vi "S4GUI.vi"(7 "Tab ObsEng":enum32{"Obs", "CCD modes", "Eng"}(tab)) -> ()   [LabVIEW 2018] (continued)
                n2555 = call "Write section_name.vi"("error in (no error)"=w5423, "section_name"="CCD_ACS3", "Channel in"=w5424) -> ("error out"=w5422:errorcluster, "Channel out"=w5427:refnum<class "Channel.lvclass">)  [unwired: 7 in]
                n2556 = call-dynamic "save config.vi"("error in (no error)"=w5422, "file config"="lastsaved.cfg", "Channel in"=w5427) -> ("error out"=w5390:errorcluster, "Channel out"=w5392:refnum<class "Channel.lvclass">)  [unwired: 7 in]
                n2557 = local read "Filter3"() -> (w5408:u8)
                n2558 = call-dynamic "Write Filter.vi"("error in (no error)"=w5390, "Filter"=w5408, "Channel in"=w5392) -> ("error out"=w5401:errorcluster, "Channel out"=w5400:refnum<class "Channel.lvclass">)  [unwired: 7 in]
                n2559 = call-dynamic "Read Interface.vi"("error in (no error)"=w5401, "Channel in"=w5400) -> ("error out"=w5403:errorcluster, "Interface.lvclass"=w5398:refnum<class "Interface.lvclass">, "Channel out"=w5399:refnum<class "Channel.lvclass">)  [unwired: 7 in]
                n2560 = call-dynamic "Write Suffix.vi"("error in (no error)"=w5403, "Suffix"=w5384, "Interface in"=w5398) -> ("error out"=w5407:errorcluster, "Interface out"=w5397:refnum<class "Interface.lvclass">)  [unwired: 7 in]
                n2561 = call-dynamic "Write ObsType.vi"("error in (no error)"=w5407, "ObsType"=w5383, "Interface in"=w5397) -> ("error out"=w5406:errorcluster, "Interface out"=w5396:refnum<class "Interface.lvclass">)  [unwired: 7 in]
                n2562 = call-dynamic "Write Object.vi"("error in (no error)"=w5406, "Object"=w5386, "Interface in"=w5396) -> ("error out"=w5405:errorcluster, "Interface out"=w5395:refnum<class "Interface.lvclass">)  [unwired: 7 in]
                n2563 = call-dynamic "Write Comments.vi"("error in (no error)"=w5405, "Comments"=w5387, "Interface in"=w5395) -> ("error out"=w5404:errorcluster, "Interface out"=w5394:refnum<class "Interface.lvclass">)  [unwired: 7 in]
                n2564 = call-dynamic "Write Observer.vi"("error in (no error)"=w5404, "Observer"=w5388, "Interface in"=w5394) -> ("error out"=w5402:errorcluster, "Interface out"=w5393:refnum<class "Interface.lvclass">)  [unwired: 7 in]
                n2565 = call-dynamic "Write Interface.vi"("error in (no error)"=w5402, "Interface.lvclass"=w5393, "Channel in"=w5399) -> ("error out"=w5389:errorcluster, "Channel out"=w5391:refnum<class "Channel.lvclass">)  [unwired: 7 in]
                n2566 = call-dynamic "Read State Machine.vi"("error in (no error)"=w5389, "Device in"=w5391) -> ("error out"=w5355:errorcluster, "State Machine.lvclass"=w5357:refnum<class "State Machine.lvclass">, "Device out"=w5428:refnum<class "Channel.lvclass">)  [unwired: 7 in]
                n2567 = call-dynamic "Read ref StatesQueue.vi"("error in (no error)"=w5355, "State Machine in"=w5357) -> ("error out"=w5362:errorcluster, "ref StatesQueue"=w5361:refnum<queue>, "State Machine out"=w5358:refnum<class "State Machine.lvclass">)  [unwired: 7 in]
                n2568 = Flush Queue(queue=w5361, error in (no error)=w5362) -> (queue out=w5363:refnum<queue>, error out=w5367:errorcluster)  [unwired: 1 out]
                n2569 = Enqueue Element(queue=w5363, element=u32 300 ("State"), error in (no error)=w5367) -> (queue out=w5364:refnum<queue>, error out=w5368:errorcluster)  [unwired: 1 in, 1 out]
                n2570 = Enqueue Element(queue=w5364, element=u32 60 ("State"), error in (no error)=w5368) -> (queue out=w5365:refnum<queue>, error out=w5366:errorcluster)  [unwired: 1 in, 1 out]
                n2571 = call-dynamic "Write ref StatesQueue.vi"("error in (no error)"=w5366, "ref StatesQueue"=w5365, "State Machine in"=w5358) -> ("error out"=w5354:errorcluster, "State Machine out"=w5356:refnum<class "State Machine.lvclass">)  [unwired: 7 in]
                n2572 = call-dynamic "Write State.vi"("error in (no error)"=w5354, "State"=0, "State Machine in"=w5356) -> ("error out"=w5420:errorcluster, "State Machine out"=w5429:refnum<class "State Machine.lvclass">)  [unwired: 7 in]
                n2573 = call-dynamic "Write State Machine.vi"("error in (no error)"=w5420, "State Machine.lvclass"=w5429, "Device in"=w5428) -> ("error out"=w5431:errorcluster, "Device out"=w5430:refnum<class "Channel.lvclass">)  [unwired: 7 in]
                n2574 = call-dynamic "Write Channel.vi"("error in (no error)"=w5431, "Channel.lvclass"=w5430, "Acquisition in"=w5413) -> ("error out"=w5409:errorcluster, "Acquisition out"=w5410:refnum<class "Acquisition.lvclass">)  [unwired: 7 in]
              }
            }
            n2575 = case shown="True" w5243 {
              tunnel: w5245 -> [w5267 w5326]
              tunnel: w5244 -> [w5266 w5325]
              tunnel: [w5267 w5324] -> w5259
              tunnel: [w5266 w5323] -> w5258
              tunnel: w5236 -> [_ w5302]
              tunnel: w5235 -> [_ w5301]
              tunnel: w5234 -> [_ w5300]
              tunnel: w5233 -> [_ w5298]
              tunnel: w5232 -> [_ w5297]
              frame False {
              }
              frame True {
                # "nome do arquivo .cfg"
                # "seção no arquivo .cfg"
                n2576 = call-dynamic "Read Channel.vi"("error in (no error)"=w5325, "Acquisition in"=w5326) -> ("error out"=w5343:errorcluster, "Channel.lvclass"=w5344:refnum<class "Channel.lvclass">, "Acquisition out"=w5345:refnum<class "Acquisition.lvclass">)  [unwired: 7 in]
                n2577 = call-dynamic "Read Interface.vi"("error in (no error)"=w5343, "Channel in"=w5344) -> ("error out"=w5295:errorcluster, "Interface.lvclass"=w5294:refnum<class "Interface.lvclass">, "Channel out"=w5291:refnum<class "Channel.lvclass">)  [unwired: 7 in]
                n2578 = call-dynamic "Write restoreExpTime.vi"("error in (no error)"=w5295, "restoreExpTime"=TRUE, "Interface in"=w5294) -> ("error out"=w5288:errorcluster, "Interface out"=w5293:refnum<class "Interface.lvclass">)  [unwired: 7 in]
                n2579 = call-dynamic "Read target cluster.vi"("error in (no error)"=w5288, "Channel in"=w5291) -> ("error out"=w5287:errorcluster, "target cluster"=w5289:T30, "Channel out"=w5290:refnum<class "Channel.lvclass">)  [unwired: 7 in]
                n2580 = stacked-sequence {
                  tunnel: w5289 -> [_ w5351]
                  tunnel: [_ w5350] -> w5285
                  tunnel: w5289 -> [w5347 _]
                  tunnel: [w5346 _] -> w5299
                  frame #0 {
                    n2581 = Unbundle By Name(w5347) -> ("FRAME_TRANSFER"=w5346:bool)
                  }
                  frame #1 {
                    # "closed"
                    n2582 = Bundle By Name(cluster=w5351, "SHUTTER_MODE"=u8 2, "FRAME_TRANSFER"=FALSE) -> (w5350:T30)
                  }
                }
                n2583 = call-dynamic "Write PREV_FT.vi"("error in (no error)"=w5287, "PREV_FT"=w5299, "Interface in"=w5293) -> ("error out"=w5286:errorcluster, "Interface out"=w5292:refnum<class "Interface.lvclass">)  [unwired: 7 in]
                n2584 = call-dynamic "Write target cluster.vi"("error in (no error)"=w5286, "target cluster"=w5285, "Channel in"=w5290) -> ("error out"=w5284:errorcluster, "Channel out"=w5283:refnum<class "Channel.lvclass">)  [unwired: 7 in]
                n2585 = Flatten To String(anything=w5285, error in (no error)=w5284) -> (data string=w5342:string, error out=w5341:errorcluster)  [unwired: 2 in, 1 out]
                n2586 = call "Write flatted cluster.vi"("error in (no error)"=w5341, "flatted cluster"=w5342, "Interface in"=w5292) -> ("error out"=w5339:errorcluster, "Interface out"=w5340:refnum<class "Interface.lvclass">)  [unwired: 7 in]
                n2587 = call-dynamic "Write Interface.vi"("error in (no error)"=w5339, "Interface.lvclass"=w5340, "Channel in"=w5283) -> ("error out"=w5335:errorcluster, "Channel out"=w5334:refnum<class "Channel.lvclass">)  [unwired: 7 in]
                n2588 = call "Write section_name.vi"("error in (no error)"=w5335, "section_name"="CCD_ACS4", "Channel in"=w5334) -> ("error out"=w5336:errorcluster, "Channel out"=w5331:refnum<class "Channel.lvclass">)  [unwired: 7 in]
                n2589 = call-dynamic "save config.vi"("error in (no error)"=w5336, "file config"="lastsaved.cfg", "Channel in"=w5331) -> ("error out"=w5305:errorcluster, "Channel out"=w5306:refnum<class "Channel.lvclass">)  [unwired: 7 in]
                n2590 = local read "Filter4"() -> (w5322:u8)
                n2591 = call-dynamic "Write Filter.vi"("error in (no error)"=w5305, "Filter"=w5322, "Channel in"=w5306) -> ("error out"=w5315:errorcluster, "Channel out"=w5314:refnum<class "Channel.lvclass">)  [unwired: 7 in]
                n2592 = call-dynamic "Read Interface.vi"("error in (no error)"=w5315, "Channel in"=w5314) -> ("error out"=w5317:errorcluster, "Interface.lvclass"=w5312:refnum<class "Interface.lvclass">, "Channel out"=w5313:refnum<class "Channel.lvclass">)  [unwired: 7 in]
                n2593 = call-dynamic "Write Suffix.vi"("error in (no error)"=w5317, "Suffix"=w5298, "Interface in"=w5312) -> ("error out"=w5321:errorcluster, "Interface out"=w5311:refnum<class "Interface.lvclass">)  [unwired: 7 in]
                n2594 = call-dynamic "Write ObsType.vi"("error in (no error)"=w5321, "ObsType"=w5297, "Interface in"=w5311) -> ("error out"=w5320:errorcluster, "Interface out"=w5310:refnum<class "Interface.lvclass">)  [unwired: 7 in]
                n2595 = call-dynamic "Write Object.vi"("error in (no error)"=w5320, "Object"=w5300, "Interface in"=w5310) -> ("error out"=w5319:errorcluster, "Interface out"=w5309:refnum<class "Interface.lvclass">)  [unwired: 7 in]
                n2596 = call-dynamic "Write Comments.vi"("error in (no error)"=w5319, "Comments"=w5301, "Interface in"=w5309) -> ("error out"=w5318:errorcluster, "Interface out"=w5308:refnum<class "Interface.lvclass">)  [unwired: 7 in]
                n2597 = call-dynamic "Write Observer.vi"("error in (no error)"=w5318, "Observer"=w5302, "Interface in"=w5308) -> ("error out"=w5316:errorcluster, "Interface out"=w5307:refnum<class "Interface.lvclass">)  [unwired: 7 in]
                n2598 = call-dynamic "Write Interface.vi"("error in (no error)"=w5316, "Interface.lvclass"=w5307, "Channel in"=w5313) -> ("error out"=w5304:errorcluster, "Channel out"=w5303:refnum<class "Channel.lvclass">)  [unwired: 7 in]
                n2599 = call-dynamic "Read State Machine.vi"("error in (no error)"=w5304, "Device in"=w5303) -> ("error out"=w5270:errorcluster, "State Machine.lvclass"=w5271:refnum<class "State Machine.lvclass">, "Device out"=w5330:refnum<class "Channel.lvclass">)  [unwired: 7 in]
                n2600 = call-dynamic "Read ref StatesQueue.vi"("error in (no error)"=w5270, "State Machine in"=w5271) -> ("error out"=w5276:errorcluster, "ref StatesQueue"=w5275:refnum<queue>, "State Machine out"=w5272:refnum<class "State Machine.lvclass">)  [unwired: 7 in]
                n2601 = Flush Queue(queue=w5275, error in (no error)=w5276) -> (queue out=w5277:refnum<queue>, error out=w5281:errorcluster)  [unwired: 1 out]
                n2602 = Enqueue Element(queue=w5277, element=u32 300 ("State"), error in (no error)=w5281) -> (queue out=w5278:refnum<queue>, error out=w5282:errorcluster)  [unwired: 1 in, 1 out]
                n2603 = Enqueue Element(queue=w5278, element=u32 60 ("State"), error in (no error)=w5282) -> (queue out=w5279:refnum<queue>, error out=w5280:errorcluster)  [unwired: 1 in, 1 out]
                n2604 = call-dynamic "Write ref StatesQueue.vi"("error in (no error)"=w5280, "ref StatesQueue"=w5279, "State Machine in"=w5272) -> ("error out"=w5269:errorcluster, "State Machine out"=w5268:refnum<class "State Machine.lvclass">)  [unwired: 7 in]
                n2605 = call-dynamic "Write State.vi"("error in (no error)"=w5269, "State"=0, "State Machine in"=w5268) -> ("error out"=w5338:errorcluster, "State Machine out"=w5329:refnum<class "State Machine.lvclass">)  [unwired: 7 in]
                n2606 = call-dynamic "Write State Machine.vi"("error in (no error)"=w5338, "State Machine.lvclass"=w5329, "Device in"=w5330) -> ("error out"=w5327:errorcluster, "Device out"=w5328:refnum<class "Channel.lvclass">)  [unwired: 7 in]
                n2607 = call-dynamic "Write Channel.vi"("error in (no error)"=w5327, "Channel.lvclass"=w5328, "Acquisition in"=w5345) -> ("error out"=w5323:errorcluster, "Acquisition out"=w5324:refnum<class "Acquisition.lvclass">)  [unwired: 7 in]
              }
            }
            n2608 = property on="Exptime ch1" class="DigNum (strict)"("Value"=w5255) -> ()  [unwired: 2 in, 2 out]
            n2609 = property on="Exptime ch2" class="DigNum (strict)"("Value"=w5255) -> ()  [unwired: 2 in, 2 out]
            n2610 = property on="Exptime ch3" class="DigNum (strict)"("Value"=w5255) -> ()  [unwired: 2 in, 2 out]
            n2611 = property on="Exptime ch4" class="DigNum (strict)"("Value"=w5255) -> ()  [unwired: 2 in, 2 out]
          }
          frame "DARK" {
            # "DARK: Shutter automatically closed and restore FRAME_TRANSFER."
            n2612 = call "Read connection.vi"("error in (no error)"=w5615, "Server in"=w5616) -> ("error out"=w5622:errorcluster, "connection"=w5621:bool, "Server out"=w5623:refnum<class "Acquisition.lvclass">)  [unwired: 7 in]
            n2613 = call "Read connection.vi"("error in (no error)"=w5619, "Server in"=w5620) -> ("error out"=w5628:errorcluster, "connection"=w5627:bool, "Server out"=w5629:refnum<class "Acquisition.lvclass">)  [unwired: 7 in]
            n2614 = call "Read connection.vi"("error in (no error)"=w5617, "Server in"=w5618) -> ("error out"=w5625:errorcluster, "connection"=w5624:bool, "Server out"=w5626:refnum<class "Acquisition.lvclass">)  [unwired: 7 in]
            n2615 = call "Read connection.vi"("error in (no error)"=w5633, "Server in"=w5634) -> ("error out"=w5631:errorcluster, "connection"=w5630:bool, "Server out"=w5632:refnum<class "Acquisition.lvclass">)  [unwired: 7 in]
            n2616 = case shown="True" w5621 {
              tunnel: w5623 -> [w5644 w5706]
              tunnel: w5622 -> [w5643 w5705]
              tunnel: [w5644 w5704] -> w5636
              tunnel: [w5643 w5703] -> w5635
              tunnel: w5614 -> [_ w5681]
              tunnel: w5613 -> [_ w5680]
              tunnel: w5612 -> [_ w5679]
              tunnel: w5611 -> [_ w5675]
              tunnel: w5610 -> [_ w5674]
              frame False {
              }
              frame True {
                # "nome do arquivo .cfg"
                # "seção no arquivo .cfg"
                # "closed"
                n2617 = call-dynamic "Read Channel.vi"("error in (no error)"=w5705, "Acquisition in"=w5706) -> ("error out"=w5723:errorcluster, "Channel.lvclass"=w5724:refnum<class "Channel.lvclass">, "Acquisition out"=w5725:refnum<class "Acquisition.lvclass">)  [unwired: 7 in]
                n2618 = call-dynamic "Read Interface.vi"("error in (no error)"=w5723, "Channel in"=w5724) -> ("error out"=w5673:errorcluster, "Interface.lvclass"=w5672:refnum<class "Interface.lvclass">, "Channel out"=w5668:refnum<class "Channel.lvclass">)  [unwired: 7 in]
                n2619 = call-dynamic "Read restoreExpTime.vi"("error in (no error)"=w5673, "Interface in"=w5672) -> ("error out"=w5670:errorcluster, "restoreExpTime"=w5669:bool, "Interface out"=w5671:refnum<class "Interface.lvclass">)  [unwired: 7 in]
                n2620 = case shown="True" w5669 {
                  tunnel: w5671 -> [w5727 w5732]
                  tunnel: w5670 -> [w5726 w5730]
                  tunnel: [w5726 w5735] -> w5677
                  tunnel: [w5727 w5734] -> w5676
                  frame False {
                  }
                  frame True {
                    n2621 = call-dynamic "Write restoreExpTime.vi"("error in (no error)"=w5730, "restoreExpTime"=FALSE, "Interface in"=w5732) -> ("error out"=w5728:errorcluster, "Interface out"=w5731:refnum<class "Interface.lvclass">)  [unwired: 7 in]
                    n2622 = call-dynamic "Read prev ExpTime.vi"("error in (no error)"=w5728, "Interface in"=w5731) -> ("error out"=w5735:errorcluster, "prev ExpTime"=w5733:dbl, "Interface out"=w5734:refnum<class "Interface.lvclass">)  [unwired: 7 in]
                    n2623 = property on="Exptime ch4" class="DigNum (strict)"("Value"=w5733) -> ()  [unwired: 2 in, 2 out]
                  }
                }
                n2624 = call-dynamic "Read PREV_FT.vi"("error in (no error)"=w5677, "Interface in"=w5676) -> ("error out"=w5667:errorcluster, "PREV_FT"=w5678:bool, "Interface out"=w5665:refnum<class "Interface.lvclass">)  [unwired: 7 in]
                n2625 = call-dynamic "Read target cluster.vi"("error in (no error)"=w5667, "Channel in"=w5668) -> ("error out"=w5662:errorcluster, "target cluster"=w5666:T30, "Channel out"=w5664:refnum<class "Channel.lvclass">)  [unwired: 7 in]
                n2626 = Bundle By Name(cluster=w5666, "SHUTTER_MODE"=u8 2, "FRAME_TRANSFER"=w5678) -> (w5663:T30)
                n2627 = call-dynamic "Write target cluster.vi"("error in (no error)"=w5662, "target cluster"=w5663, "Channel in"=w5664) -> ("error out"=w5661:errorcluster, "Channel out"=w5660:refnum<class "Channel.lvclass">)  [unwired: 7 in]
                n2628 = Flatten To String(anything=w5663, error in (no error)=w5661) -> (data string=w5722:string, error out=w5721:errorcluster)  [unwired: 2 in, 1 out]
                n2629 = call "Write flatted cluster.vi"("error in (no error)"=w5721, "flatted cluster"=w5722, "Interface in"=w5665) -> ("error out"=w5718:errorcluster, "Interface out"=w5719:refnum<class "Interface.lvclass">)  [unwired: 7 in]
                n2630 = call-dynamic "Write Interface.vi"("error in (no error)"=w5718, "Interface.lvclass"=w5719, "Channel in"=w5660) -> ("error out"=w5714:errorcluster, "Channel out"=w5713:refnum<class "Channel.lvclass">)  [unwired: 7 in]
                n2631 = call "Write section_name.vi"("error in (no error)"=w5714, "section_name"="CCD_ACS4", "Channel in"=w5713) -> ("error out"=w5715:errorcluster, "Channel out"=w5710:refnum<class "Channel.lvclass">)  [unwired: 7 in]
                n2632 = call-dynamic "save config.vi"("error in (no error)"=w5715, "file config"="lastsaved.cfg", "Channel in"=w5710) -> ("error out"=w5684:errorcluster, "Channel out"=w5685:refnum<class "Channel.lvclass">)  [unwired: 7 in]
                n2633 = local read "Filter4"() -> (w5686:u8)
                n2634 = call-dynamic "Write Filter.vi"("error in (no error)"=w5684, "Filter"=w5686, "Channel in"=w5685) -> ("error out"=w5693:errorcluster, "Channel out"=w5694:refnum<class "Channel.lvclass">)  [unwired: 7 in]
                n2635 = call-dynamic "Read Interface.vi"("error in (no error)"=w5693, "Channel in"=w5694) -> ("error out"=w5691:errorcluster, "Interface.lvclass"=w5696:refnum<class "Interface.lvclass">, "Channel out"=w5695:refnum<class "Channel.lvclass">)  [unwired: 7 in]
                n2636 = call-dynamic "Write Suffix.vi"("error in (no error)"=w5691, "Suffix"=w5675, "Interface in"=w5696) -> ("error out"=w5687:errorcluster, "Interface out"=w5697:refnum<class "Interface.lvclass">)  [unwired: 7 in]
                n2637 = call-dynamic "Write ObsType.vi"("error in (no error)"=w5687, "ObsType"=w5674, "Interface in"=w5697) -> ("error out"=w5688:errorcluster, "Interface out"=w5698:refnum<class "Interface.lvclass">)  [unwired: 7 in]
                n2638 = call-dynamic "Write Object.vi"("error in (no error)"=w5688, "Object"=w5681, "Interface in"=w5698) -> ("error out"=w5689:errorcluster, "Interface out"=w5699:refnum<class "Interface.lvclass">)  [unwired: 7 in]
                n2639 = call-dynamic "Write Comments.vi"("error in (no error)"=w5689, "Comments"=w5680, "Interface in"=w5699) -> ("error out"=w5690:errorcluster, "Interface out"=w5700:refnum<class "Interface.lvclass">)  [unwired: 7 in]
                n2640 = call-dynamic "Write Observer.vi"("error in (no error)"=w5690, "Observer"=w5679, "Interface in"=w5700) -> ("error out"=w5692:errorcluster, "Interface out"=w5701:refnum<class "Interface.lvclass">)  [unwired: 7 in]
                n2641 = call-dynamic "Write Interface.vi"("error in (no error)"=w5692, "Interface.lvclass"=w5701, "Channel in"=w5695) -> ("error out"=w5682:errorcluster, "Channel out"=w5683:refnum<class "Channel.lvclass">)  [unwired: 7 in]
                n2642 = call-dynamic "Read State Machine.vi"("error in (no error)"=w5682, "Device in"=w5683) -> ("error out"=w5647:errorcluster, "State Machine.lvclass"=w5648:refnum<class "State Machine.lvclass">, "Device out"=w5709:refnum<class "Channel.lvclass">)  [unwired: 7 in]
                n2643 = call-dynamic "Read ref StatesQueue.vi"("error in (no error)"=w5647, "State Machine in"=w5648) -> ("error out"=w5658:errorcluster, "ref StatesQueue"=w5650:refnum<queue>, "State Machine out"=w5659:refnum<class "State Machine.lvclass">)  [unwired: 7 in]
                n2644 = Flush Queue(queue=w5650, error in (no error)=w5658) -> (queue out=w5649:refnum<queue>, error out=w5654:errorcluster)  [unwired: 1 out]
                n2645 = Enqueue Element(queue=w5649, element=u32 300 ("State"), error in (no error)=w5654) -> (queue out=w5657:refnum<queue>, error out=w5653:errorcluster)  [unwired: 1 in, 1 out]
                n2646 = Enqueue Element(queue=w5657, element=u32 60 ("State"), error in (no error)=w5653) -> (queue out=w5656:refnum<queue>, error out=w5655:errorcluster)  [unwired: 1 in, 1 out]
                n2647 = call-dynamic "Write ref StatesQueue.vi"("error in (no error)"=w5655, "ref StatesQueue"=w5656, "State Machine in"=w5659) -> ("error out"=w5645:errorcluster, "State Machine out"=w5646:refnum<class "State Machine.lvclass">)  [unwired: 7 in]
                n2648 = call-dynamic "Write State.vi"("error in (no error)"=w5645, "State"=0, "State Machine in"=w5646) -> ("error out"=w5717:errorcluster, "State Machine out"=w5708:refnum<class "State Machine.lvclass">)  [unwired: 7 in]
                n2649 = call-dynamic "Write State Machine.vi"("error in (no error)"=w5717, "State Machine.lvclass"=w5708, "Device in"=w5709) -> ("error out"=w5707:errorcluster, "Device out"=w5702:refnum<class "Channel.lvclass">)  [unwired: 7 in]
                n2650 = call-dynamic "Write Channel.vi"("error in (no error)"=w5707, "Channel.lvclass"=w5702, "Acquisition in"=w5725) -> ("error out"=w5703:errorcluster, "Acquisition out"=w5704:refnum<class "Acquisition.lvclass">)  [unwired: 7 in]
              }
            }
            n2651 = case shown="True" w5627 {
              tunnel: w5629 -> [w5830 w5891]
              tunnel: w5628 -> [w5829 w5890]
              tunnel: [w5830 w5889] -> w5640
              tunnel: [w5829 w5888] -> w5639
              tunnel: w5614 -> [_ w5867]
              tunnel: w5613 -> [_ w5866]
              tunnel: w5612 -> [_ w5865]
              tunnel: w5611 -> [_ w5861]
              tunnel: w5610 -> [_ w5860]
              frame False {
              }
              frame True {
                # "nome do arquivo .cfg"
                # "seção no arquivo .cfg"
                # "closed"
                n2652 = call-dynamic "Read Channel.vi"("error in (no error)"=w5890, "Acquisition in"=w5891) -> ("error out"=w5894:errorcluster, "Channel.lvclass"=w5893:refnum<class "Channel.lvclass">, "Acquisition out"=w5892:refnum<class "Acquisition.lvclass">)  [unwired: 7 in]
                n2653 = call-dynamic "Read Interface.vi"("error in (no error)"=w5894, "Channel in"=w5893) -> ("error out"=w5859:errorcluster, "Interface.lvclass"=w5858:refnum<class "Interface.lvclass">, "Channel out"=w5854:refnum<class "Channel.lvclass">)  [unwired: 7 in]
                n2654 = call-dynamic "Read restoreExpTime.vi"("error in (no error)"=w5859, "Interface in"=w5858) -> ("error out"=w5856:errorcluster, "restoreExpTime"=w5855:bool, "Interface out"=w5857:refnum<class "Interface.lvclass">)  [unwired: 7 in]
                n2655 = case shown="True" w5855 {
                  tunnel: w5857 -> [w5913 w5918]
                  tunnel: [w5913 w5921] -> w5863
                  tunnel: w5856 -> [w5912 w5916]
                  tunnel: [w5912 w5920] -> w5862
                  frame False {
                  }
                  frame True {
                    n2656 = call-dynamic "Write restoreExpTime.vi"("error in (no error)"=w5916, "restoreExpTime"=FALSE, "Interface in"=w5918) -> ("error out"=w5915:errorcluster, "Interface out"=w5917:refnum<class "Interface.lvclass">)  [unwired: 7 in]
                    n2657 = call-dynamic "Read prev ExpTime.vi"("error in (no error)"=w5915, "Interface in"=w5917) -> ("error out"=w5920:errorcluster, "prev ExpTime"=w5919:dbl, "Interface out"=w5921:refnum<class "Interface.lvclass">)  [unwired: 7 in]
                    n2658 = property on="Exptime ch2" class="DigNum (strict)"("Value"=w5919) -> ()  [unwired: 2 in, 2 out]
                  }
                }
                n2659 = call-dynamic "Read PREV_FT.vi"("error in (no error)"=w5862, "Interface in"=w5863) -> ("error out"=w5853:errorcluster, "PREV_FT"=w5864:bool, "Interface out"=w5851:refnum<class "Interface.lvclass">)  [unwired: 7 in]
                n2660 = call-dynamic "Read target cluster.vi"("error in (no error)"=w5853, "Channel in"=w5854) -> ("error out"=w5848:errorcluster, "target cluster"=w5852:T30, "Channel out"=w5850:refnum<class "Channel.lvclass">)  [unwired: 7 in]
                n2661 = Bundle By Name(cluster=w5852, "SHUTTER_MODE"=u8 2, "FRAME_TRANSFER"=w5864) -> (w5849:T30)
                n2662 = call-dynamic "Write target cluster.vi"("error in (no error)"=w5848, "target cluster"=w5849, "Channel in"=w5850) -> ("error out"=w5847:errorcluster, "Channel out"=w5846:refnum<class "Channel.lvclass">)  [unwired: 7 in]
                n2663 = Flatten To String(anything=w5849, error in (no error)=w5847) -> (data string=w5895:string, error out=w5896:errorcluster)  [unwired: 2 in, 1 out]
                n2664 = call "Write flatted cluster.vi"("error in (no error)"=w5896, "flatted cluster"=w5895, "Interface in"=w5851) -> ("error out"=w5899:errorcluster, "Interface out"=w5898:refnum<class "Interface.lvclass">)  [unwired: 7 in]
                n2665 = call-dynamic "Write Interface.vi"("error in (no error)"=w5899, "Interface.lvclass"=w5898, "Channel in"=w5846) -> ("error out"=w5903:errorcluster, "Channel out"=w5904:refnum<class "Channel.lvclass">)  [unwired: 7 in]
                n2666 = call "Write section_name.vi"("error in (no error)"=w5903, "section_name"="CCD_ACS2", "Channel in"=w5904) -> ("error out"=w5902:errorcluster, "Channel out"=w5907:refnum<class "Channel.lvclass">)  [unwired: 7 in]
                n2667 = call-dynamic "save config.vi"("error in (no error)"=w5902, "file config"="lastsaved.cfg", "Channel in"=w5907) -> ("error out"=w5870:errorcluster, "Channel out"=w5871:refnum<class "Channel.lvclass">)  [unwired: 7 in]
                n2668 = local read "Filter2"() -> (w5872:u8)
                n2669 = call-dynamic "Write Filter.vi"("error in (no error)"=w5870, "Filter"=w5872, "Channel in"=w5871) -> ("error out"=w5879:errorcluster, "Channel out"=w5880:refnum<class "Channel.lvclass">)  [unwired: 7 in]
                n2670 = call-dynamic "Read Interface.vi"("error in (no error)"=w5879, "Channel in"=w5880) -> ("error out"=w5877:errorcluster, "Interface.lvclass"=w5882:refnum<class "Interface.lvclass">, "Channel out"=w5881:refnum<class "Channel.lvclass">)  [unwired: 7 in]
                n2671 = call-dynamic "Write Suffix.vi"("error in (no error)"=w5877, "Suffix"=w5861, "Interface in"=w5882) -> ("error out"=w5873:errorcluster, "Interface out"=w5883:refnum<class "Interface.lvclass">)  [unwired: 7 in]
                n2672 = call-dynamic "Write ObsType.vi"("error in (no error)"=w5873, "ObsType"=w5860, "Interface in"=w5883) -> ("error out"=w5874:errorcluster, "Interface out"=w5884:refnum<class "Interface.lvclass">)  [unwired: 7 in]
                n2673 = call-dynamic "Write Object.vi"("error in (no error)"=w5874, "Object"=w5867, "Interface in"=w5884) -> ("error out"=w5875:errorcluster, "Interface out"=w5885:refnum<class "Interface.lvclass">)  [unwired: 7 in]
                n2674 = call-dynamic "Write Comments.vi"("error in (no error)"=w5875, "Comments"=w5866, "Interface in"=w5885) -> ("error out"=w5876:errorcluster, "Interface out"=w5886:refnum<class "Interface.lvclass">)  [unwired: 7 in]
                n2675 = call-dynamic "Write Observer.vi"("error in (no error)"=w5876, "Observer"=w5865, "Interface in"=w5886) -> ("error out"=w5878:errorcluster, "Interface out"=w5887:refnum<class "Interface.lvclass">)  [unwired: 7 in]
                n2676 = call-dynamic "Write Interface.vi"("error in (no error)"=w5878, "Interface.lvclass"=w5887, "Channel in"=w5881) -> ("error out"=w5868:errorcluster, "Channel out"=w5869:refnum<class "Channel.lvclass">)  [unwired: 7 in]
                n2677 = call-dynamic "Read State Machine.vi"("error in (no error)"=w5868, "Device in"=w5869) -> ("error out"=w5835:errorcluster, "State Machine.lvclass"=w5836:refnum<class "State Machine.lvclass">, "Device out"=w5908:refnum<class "Channel.lvclass">)  [unwired: 7 in]
                n2678 = call-dynamic "Read ref StatesQueue.vi"("error in (no error)"=w5835, "State Machine in"=w5836) -> ("error out"=w5844:errorcluster, "ref StatesQueue"=w5834:refnum<queue>, "State Machine out"=w5845:refnum<class "State Machine.lvclass">)  [unwired: 7 in]
                n2679 = Flush Queue(queue=w5834, error in (no error)=w5844) -> (queue out=w5833:refnum<queue>, error out=w5840:errorcluster)  [unwired: 1 out]
                n2680 = Enqueue Element(queue=w5833, element=u32 300 ("State"), error in (no error)=w5840) -> (queue out=w5843:refnum<queue>, error out=w5839:errorcluster)  [unwired: 1 in, 1 out]
                n2681 = Enqueue Element(queue=w5843, element=u32 60 ("State"), error in (no error)=w5839) -> (queue out=w5842:refnum<queue>, error out=w5841:errorcluster)  [unwired: 1 in, 1 out]
                n2682 = call-dynamic "Write ref StatesQueue.vi"("error in (no error)"=w5841, "ref StatesQueue"=w5842, "State Machine in"=w5845) -> ("error out"=w5831:errorcluster, "State Machine out"=w5832:refnum<class "State Machine.lvclass">)  [unwired: 7 in]
                n2683 = call-dynamic "Write State.vi"("error in (no error)"=w5831, "State"=0, "State Machine in"=w5832) -> ("error out"=w5900:errorcluster, "State Machine out"=w5909:refnum<class "State Machine.lvclass">)  [unwired: 7 in]
                n2684 = call-dynamic "Write State Machine.vi"("error in (no error)"=w5900, "State Machine.lvclass"=w5909, "Device in"=w5908) -> ("error out"=w5911:errorcluster, "Device out"=w5910:refnum<class "Channel.lvclass">)  [unwired: 7 in]
                n2685 = call-dynamic "Write Channel.vi"("error in (no error)"=w5911, "Channel.lvclass"=w5910, "Acquisition in"=w5892) -> ("error out"=w5888:errorcluster, "Acquisition out"=w5889:refnum<class "Acquisition.lvclass">)  [unwired: 7 in]
              }
            }
            n2686 = case shown="True" w5624 {
              tunnel: w5626 -> [w5737 w5798]
              tunnel: w5625 -> [w5736 w5797]
              tunnel: [w5737 w5796] -> w5638
              tunnel: [w5736 w5795] -> w5637
              tunnel: w5614 -> [_ w5774]
              tunnel: w5613 -> [_ w5773]
              tunnel: w5612 -> [_ w5772]
              tunnel: w5611 -> [_ w5768]
              tunnel: w5610 -> [_ w5767]
              frame False {
              }
              frame True {
                # "nome do arquivo .cfg"
                # "seção no arquivo .cfg"
                # "closed"
                n2687 = call-dynamic "Read Channel.vi"("error in (no error)"=w5797, "Acquisition in"=w5798) -> ("error out"=w5801:errorcluster, "Channel.lvclass"=w5800:refnum<class "Channel.lvclass">, "Acquisition out"=w5799:refnum<class "Acquisition.lvclass">)  [unwired: 7 in]
                n2688 = call-dynamic "Read Interface.vi"("error in (no error)"=w5801, "Channel in"=w5800) -> ("error out"=w5764:errorcluster, "Interface.lvclass"=w5766:refnum<class "Interface.lvclass">, "Channel out"=w5761:refnum<class "Channel.lvclass">)  [unwired: 7 in]
                n2689 = call-dynamic "Read restoreExpTime.vi"("error in (no error)"=w5764, "Interface in"=w5766) -> ("error out"=w5763:errorcluster, "restoreExpTime"=w5762:bool, "Interface out"=w5765:refnum<class "Interface.lvclass">)  [unwired: 7 in]
                n2690 = case shown="True" w5762 {
                  tunnel: w5765 -> [w5820 w5825]
                  tunnel: [w5820 w5828] -> w5770
                  tunnel: w5763 -> [w5819 w5824]
                  tunnel: [w5819 w5827] -> w5769
                  frame False {
                  }
                  frame True {
                    n2691 = call-dynamic "Write restoreExpTime.vi"("error in (no error)"=w5824, "restoreExpTime"=FALSE, "Interface in"=w5825) -> ("error out"=w5821:errorcluster, "Interface out"=w5822:refnum<class "Interface.lvclass">)  [unwired: 7 in]
                    n2692 = call-dynamic "Read prev ExpTime.vi"("error in (no error)"=w5821, "Interface in"=w5822) -> ("error out"=w5827:errorcluster, "prev ExpTime"=w5826:dbl, "Interface out"=w5828:refnum<class "Interface.lvclass">)  [unwired: 7 in]
                    n2693 = property on="Exptime ch3" class="DigNum (strict)"("Value"=w5826) -> ()  [unwired: 2 in, 2 out]
                  }
                }
                n2694 = call-dynamic "Read PREV_FT.vi"("error in (no error)"=w5769, "Interface in"=w5770) -> ("error out"=w5760:errorcluster, "PREV_FT"=w5771:bool, "Interface out"=w5758:refnum<class "Interface.lvclass">)  [unwired: 7 in]
                n2695 = call-dynamic "Read target cluster.vi"("error in (no error)"=w5760, "Channel in"=w5761) -> ("error out"=w5755:errorcluster, "target cluster"=w5759:T30, "Channel out"=w5757:refnum<class "Channel.lvclass">)  [unwired: 7 in]
                n2696 = Bundle By Name(cluster=w5759, "SHUTTER_MODE"=u8 2, "FRAME_TRANSFER"=w5771) -> (w5756:T30)
                n2697 = call-dynamic "Write target cluster.vi"("error in (no error)"=w5755, "target cluster"=w5756, "Channel in"=w5757) -> ("error out"=w5754:errorcluster, "Channel out"=w5753:refnum<class "Channel.lvclass">)  [unwired: 7 in]
                n2698 = Flatten To String(anything=w5756, error in (no error)=w5754) -> (data string=w5802:string, error out=w5803:errorcluster)  [unwired: 2 in, 1 out]
                n2699 = call "Write flatted cluster.vi"("error in (no error)"=w5803, "flatted cluster"=w5802, "Interface in"=w5758) -> ("error out"=w5806:errorcluster, "Interface out"=w5805:refnum<class "Interface.lvclass">)  [unwired: 7 in]
                n2700 = call-dynamic "Write Interface.vi"("error in (no error)"=w5806, "Interface.lvclass"=w5805, "Channel in"=w5753) -> ("error out"=w5810:errorcluster, "Channel out"=w5811:refnum<class "Channel.lvclass">)  [unwired: 7 in]
                n2701 = call "Write section_name.vi"("error in (no error)"=w5810, "section_name"="CCD_ACS3", "Channel in"=w5811) -> ("error out"=w5809:errorcluster, "Channel out"=w5814:refnum<class "Channel.lvclass">)  [unwired: 7 in]
                n2702 = call-dynamic "save config.vi"("error in (no error)"=w5809, "file config"="lastsaved.cfg", "Channel in"=w5814) -> ("error out"=w5777:errorcluster, "Channel out"=w5778:refnum<class "Channel.lvclass">)  [unwired: 7 in]
                n2703 = local read "Filter3"() -> (w5779:u8)
                n2704 = call-dynamic "Write Filter.vi"("error in (no error)"=w5777, "Filter"=w5779, "Channel in"=w5778) -> ("error out"=w5786:errorcluster, "Channel out"=w5787:refnum<class "Channel.lvclass">)  [unwired: 7 in]
                n2705 = call-dynamic "Read Interface.vi"("error in (no error)"=w5786, "Channel in"=w5787) -> ("error out"=w5784:errorcluster, "Interface.lvclass"=w5789:refnum<class "Interface.lvclass">, "Channel out"=w5788:refnum<class "Channel.lvclass">)  [unwired: 7 in]
                n2706 = call-dynamic "Write Suffix.vi"("error in (no error)"=w5784, "Suffix"=w5768, "Interface in"=w5789) -> ("error out"=w5780:errorcluster, "Interface out"=w5790:refnum<class "Interface.lvclass">)  [unwired: 7 in]
                n2707 = call-dynamic "Write ObsType.vi"("error in (no error)"=w5780, "ObsType"=w5767, "Interface in"=w5790) -> ("error out"=w5781:errorcluster, "Interface out"=w5791:refnum<class "Interface.lvclass">)  [unwired: 7 in]
                n2708 = call-dynamic "Write Object.vi"("error in (no error)"=w5781, "Object"=w5774, "Interface in"=w5791) -> ("error out"=w5782:errorcluster, "Interface out"=w5792:refnum<class "Interface.lvclass">)  [unwired: 7 in]
                n2709 = call-dynamic "Write Comments.vi"("error in (no error)"=w5782, "Comments"=w5773, "Interface in"=w5792) -> ("error out"=w5783:errorcluster, "Interface out"=w5793:refnum<class "Interface.lvclass">)  [unwired: 7 in]
                n2710 = call-dynamic "Write Observer.vi"("error in (no error)"=w5783, "Observer"=w5772, "Interface in"=w5793) -> ("error out"=w5785:errorcluster, "Interface out"=w5794:refnum<class "Interface.lvclass">)  [unwired: 7 in]
                n2711 = call-dynamic "Write Interface.vi"("error in (no error)"=w5785, "Interface.lvclass"=w5794, "Channel in"=w5788) -> ("error out"=w5775:errorcluster, "Channel out"=w5776:refnum<class "Channel.lvclass">)  [unwired: 7 in]
                n2712 = call-dynamic "Read State Machine.vi"("error in (no error)"=w5775, "Device in"=w5776) -> ("error out"=w5741:errorcluster, "State Machine.lvclass"=w5740:refnum<class "State Machine.lvclass">, "Device out"=w5815:refnum<class "Channel.lvclass">)  [unwired: 7 in]
                n2713 = call-dynamic "Read ref StatesQueue.vi"("error in (no error)"=w5741, "State Machine in"=w5740) -> ("error out"=w5751:errorcluster, "ref StatesQueue"=w5743:refnum<queue>, "State Machine out"=w5752:refnum<class "State Machine.lvclass">)  [unwired: 7 in]
                n2714 = Flush Queue(queue=w5743, error in (no error)=w5751) -> (queue out=w5742:refnum<queue>, error out=w5747:errorcluster)  [unwired: 1 out]
                n2715 = Enqueue Element(queue=w5742, element=u32 300 ("State"), error in (no error)=w5747) -> (queue out=w5750:refnum<queue>, error out=w5746:errorcluster)  [unwired: 1 in, 1 out]
                n2716 = Enqueue Element(queue=w5750, element=u32 60 ("State"), error in (no error)=w5746) -> (queue out=w5749:refnum<queue>, error out=w5748:errorcluster)  [unwired: 1 in, 1 out]
                n2717 = call-dynamic "Write ref StatesQueue.vi"("error in (no error)"=w5748, "ref StatesQueue"=w5749, "State Machine in"=w5752) -> ("error out"=w5738:errorcluster, "State Machine out"=w5739:refnum<class "State Machine.lvclass">)  [unwired: 7 in]
                n2718 = call-dynamic "Write State.vi"("error in (no error)"=w5738, "State"=0, "State Machine in"=w5739) -> ("error out"=w5807:errorcluster, "State Machine out"=w5816:refnum<class "State Machine.lvclass">)  [unwired: 7 in]
                n2719 = call-dynamic "Write State Machine.vi"("error in (no error)"=w5807, "State Machine.lvclass"=w5816, "Device in"=w5815) -> ("error out"=w5818:errorcluster, "Device out"=w5817:refnum<class "Channel.lvclass">)  [unwired: 7 in]
                n2720 = call-dynamic "Write Channel.vi"("error in (no error)"=w5818, "Channel.lvclass"=w5817, "Acquisition in"=w5799) -> ("error out"=w5795:errorcluster, "Acquisition out"=w5796:refnum<class "Acquisition.lvclass">)  [unwired: 7 in]
              }
            }
            n2721 = case shown="True" w5630 {
              tunnel: [w5922 w6001] -> w5641
              tunnel: [w5923 w6000] -> w5642
              tunnel: w5632 -> [w5923 w5982]
              tunnel: w5631 -> [w5922 w5981]
              tunnel: w5614 -> [_ w5960]
              tunnel: w5613 -> [_ w5959]
              tunnel: w5612 -> [_ w5958]
              tunnel: w5611 -> [_ w5954]
              tunnel: w5610 -> [_ w5953]
              frame False {
              }
              frame True {
                # "nome do arquivo .cfg"
                # "seção no arquivo .cfg"
                # "closed"
                n2722 = call-dynamic "Read Channel.vi"("error in (no error)"=w5981, "Acquisition in"=w5982) -> ("error out"=w6002:errorcluster, "Channel.lvclass"=w6003:refnum<class "Channel.lvclass">, "Acquisition out"=w6004:refnum<class "Acquisition.lvclass">)  [unwired: 7 in]
                n2723 = call-dynamic "Read Interface.vi"("error in (no error)"=w6002, "Channel in"=w6003) -> ("error out"=w5951:errorcluster, "Interface.lvclass"=w5952:refnum<class "Interface.lvclass">, "Channel out"=w5947:refnum<class "Channel.lvclass">)  [unwired: 7 in]
                n2724 = call-dynamic "Read restoreExpTime.vi"("error in (no error)"=w5951, "Interface in"=w5952) -> ("error out"=w5949:errorcluster, "restoreExpTime"=w5948:bool, "Interface out"=w5950:refnum<class "Interface.lvclass">)  [unwired: 7 in]
                n2725 = case shown="True" w5948 {
                  tunnel: [w6006 w6014] -> w5956
                  tunnel: [w6005 w6013] -> w5955
                  tunnel: w5950 -> [w6006 w6011]
                  tunnel: w5949 -> [w6005 w6009]
                  frame False {
                  }
                  frame True {
                    n2726 = call-dynamic "Write restoreExpTime.vi"("error in (no error)"=w6009, "restoreExpTime"=FALSE, "Interface in"=w6011) -> ("error out"=w6008:errorcluster, "Interface out"=w6010:refnum<class "Interface.lvclass">)  [unwired: 7 in]
                    n2727 = call-dynamic "Read prev ExpTime.vi"("error in (no error)"=w6008, "Interface in"=w6010) -> ("error out"=w6013:errorcluster, "prev ExpTime"=w6012:dbl, "Interface out"=w6014:refnum<class "Interface.lvclass">)  [unwired: 7 in]
                    n2728 = property on="Exptime ch1" class="DigNum (strict)"("Value"=w6012) -> ()  [unwired: 2 in, 2 out]
                  }
                }
                n2729 = call-dynamic "Read PREV_FT.vi"("error in (no error)"=w5955, "Interface in"=w5956) -> ("error out"=w5944:errorcluster, "PREV_FT"=w5957:bool, "Interface out"=w5939:refnum<class "Interface.lvclass">)  [unwired: 7 in]
                n2730 = call-dynamic "Read target cluster.vi"("error in (no error)"=w5944, "Channel in"=w5947) -> ("error out"=w5943:errorcluster, "target cluster"=w5941:T30, "Channel out"=w5946:refnum<class "Channel.lvclass">)  [unwired: 7 in]
                n2731 = Bundle By Name(cluster=w5941, "SHUTTER_MODE"=u8 2, "FRAME_TRANSFER"=w5957) -> (w5940:T30)
                n2732 = call-dynamic "Write target cluster.vi"("error in (no error)"=w5943, "target cluster"=w5940, "Channel in"=w5946) -> ("error out"=w5942:errorcluster, "Channel out"=w5945:refnum<class "Channel.lvclass">)  [unwired: 7 in]
                n2733 = Flatten To String(anything=w5940, error in (no error)=w5942) -> (data string=w5999:string, error out=w5998:errorcluster)  [unwired: 2 in, 1 out]
                n2734 = call "Write flatted cluster.vi"("error in (no error)"=w5998, "flatted cluster"=w5999, "Interface in"=w5939) -> ("error out"=w5995:errorcluster, "Interface out"=w5996:refnum<class "Interface.lvclass">)  [unwired: 7 in]
                n2735 = call-dynamic "Write Interface.vi"("error in (no error)"=w5995, "Interface.lvclass"=w5996, "Channel in"=w5945) -> ("error out"=w5991:errorcluster, "Channel out"=w5990:refnum<class "Channel.lvclass">)  [unwired: 7 in]
                n2736 = call "Write section_name.vi"("error in (no error)"=w5991, "section_name"="CCD_ACS1", "Channel in"=w5990) -> ("error out"=w5992:errorcluster, "Channel out"=w5987:refnum<class "Channel.lvclass">)  [unwired: 7 in]
                n2737 = call-dynamic "save config.vi"("error in (no error)"=w5992, "file config"="lastsaved.cfg", "Channel in"=w5987) -> ("error out"=w5963:errorcluster, "Channel out"=w5964:refnum<class "Channel.lvclass">)  [unwired: 7 in]
                n2738 = local read "Filter1"() -> (w5965:u8)
                n2739 = call-dynamic "Write Filter.vi"("error in (no error)"=w5963, "Filter"=w5965, "Channel in"=w5964) -> ("error out"=w5972:errorcluster, "Channel out"=w5973:refnum<class "Channel.lvclass">)  [unwired: 7 in]
                n2740 = call-dynamic "Read Interface.vi"("error in (no error)"=w5972, "Channel in"=w5973) -> ("error out"=w5970:errorcluster, "Interface.lvclass"=w5975:refnum<class "Interface.lvclass">, "Channel out"=w5974:refnum<class "Channel.lvclass">)  [unwired: 7 in]
                n2741 = call-dynamic "Write Suffix.vi"("error in (no error)"=w5970, "Suffix"=w5954, "Interface in"=w5975) -> ("error out"=w5966:errorcluster, "Interface out"=w5976:refnum<class "Interface.lvclass">)  [unwired: 7 in]
                n2742 = call-dynamic "Write ObsType.vi"("error in (no error)"=w5966, "ObsType"=w5953, "Interface in"=w5976) -> ("error out"=w5967:errorcluster, "Interface out"=w5977:refnum<class "Interface.lvclass">)  [unwired: 7 in]
                n2743 = call-dynamic "Write Object.vi"("error in (no error)"=w5967, "Object"=w5960, "Interface in"=w5977) -> ("error out"=w5968:errorcluster, "Interface out"=w5978:refnum<class "Interface.lvclass">)  [unwired: 7 in]
                n2744 = call-dynamic "Write Comments.vi"("error in (no error)"=w5968, "Comments"=w5959, "Interface in"=w5978) -> ("error out"=w5969:errorcluster, "Interface out"=w5979:refnum<class "Interface.lvclass">)  [unwired: 7 in]
                n2745 = call-dynamic "Write Observer.vi"("error in (no error)"=w5969, "Observer"=w5958, "Interface in"=w5979) -> ("error out"=w5971:errorcluster, "Interface out"=w5980:refnum<class "Interface.lvclass">)  [unwired: 7 in]
                n2746 = call-dynamic "Write Interface.vi"("error in (no error)"=w5971, "Interface.lvclass"=w5980, "Channel in"=w5974) -> ("error out"=w5961:errorcluster, "Channel out"=w5962:refnum<class "Channel.lvclass">)  [unwired: 7 in]
                n2747 = call-dynamic "Read State Machine.vi"("error in (no error)"=w5961, "Device in"=w5962) -> ("error out"=w5927:errorcluster, "State Machine.lvclass"=w5929:refnum<class "State Machine.lvclass">, "Device out"=w5986:refnum<class "Channel.lvclass">)  [unwired: 7 in]
                n2748 = call-dynamic "Read ref StatesQueue.vi"("error in (no error)"=w5927, "State Machine in"=w5929) -> ("error out"=w5937:errorcluster, "ref StatesQueue"=w5925:refnum<queue>, "State Machine out"=w5938:refnum<class "State Machine.lvclass">)  [unwired: 7 in]
                n2749 = Flush Queue(queue=w5925, error in (no error)=w5937) -> (queue out=w5924:refnum<queue>, error out=w5933:errorcluster)  [unwired: 1 out]
                n2750 = Enqueue Element(queue=w5924, element=u32 300 ("State"), error in (no error)=w5933) -> (queue out=w5936:refnum<queue>, error out=w5932:errorcluster)  [unwired: 1 in, 1 out]
                n2751 = Enqueue Element(queue=w5936, element=u32 60 ("State"), error in (no error)=w5932) -> (queue out=w5935:refnum<queue>, error out=w5934:errorcluster)  [unwired: 1 in, 1 out]
                n2752 = call-dynamic "Write ref StatesQueue.vi"("error in (no error)"=w5934, "ref StatesQueue"=w5935, "State Machine in"=w5938) -> ("error out"=w5926:errorcluster, "State Machine out"=w5928:refnum<class "State Machine.lvclass">)  [unwired: 7 in]
                n2753 = call-dynamic "Write State.vi"("error in (no error)"=w5926, "State"=0, "State Machine in"=w5928) -> ("error out"=w5994:errorcluster, "State Machine out"=w5985:refnum<class "State Machine.lvclass">)  [unwired: 7 in]
                n2754 = call-dynamic "Write State Machine.vi"("error in (no error)"=w5994, "State Machine.lvclass"=w5985, "Device in"=w5986) -> ("error out"=w5983:errorcluster, "Device out"=w5984:refnum<class "Channel.lvclass">)  [unwired: 7 in]
                n2755 = call-dynamic "Write Channel.vi"("error in (no error)"=w5983, "Channel.lvclass"=w5984, "Acquisition in"=w6004) -> ("error out"=w6001:errorcluster, "Acquisition out"=w6000:refnum<class "Acquisition.lvclass">)  [unwired: 7 in]
              }
            }
          }
          frame "OBJECT", Default {
            # "OBJECT, DFLAT,SFLAT and FOCUS: Shutter automatically open and restore FRAME_TRANSFER."
            n2756 = call "Read connection.vi"("error in (no error)"=w6038, "Server in"=w6039) -> ("error out"=w6036:errorcluster, "connection"=w6035:bool, "Server out"=w6037:refnum<class "Acquisition.lvclass">)  [unwired: 7 in]
            n2757 = call "Read connection.vi"("error in (no error)"=w6020, "Server in"=w6021) -> ("error out"=w6027:errorcluster, "connection"=w6026:bool, "Server out"=w6028:refnum<class "Acquisition.lvclass">)  [unwired: 7 in]
            n2758 = call "Read connection.vi"("error in (no error)"=w6022, "Server in"=w6023) -> ("error out"=w6030:errorcluster, "connection"=w6029:bool, "Server out"=w6031:refnum<class "Acquisition.lvclass">)  [unwired: 7 in]
            n2759 = call "Read connection.vi"("error in (no error)"=w6024, "Server in"=w6025) -> ("error out"=w6033:errorcluster, "connection"=w6032:bool, "Server out"=w6034:refnum<class "Acquisition.lvclass">)  [unwired: 7 in]
            n2760 = case shown="True" w6026 {
              tunnel: w6028 -> [w6049 w6116]
              tunnel: w6027 -> [w6048 w6115]
              tunnel: [w6049 w6114] -> w6041
              tunnel: [w6048 w6113] -> w6040
              tunnel: w6019 -> [_ w6097]
              tunnel: w6018 -> [_ w6096]
              tunnel: w6017 -> [_ w6095]
              tunnel: w6016 -> [_ w6091]
              tunnel: w6015 -> [_ w6090]
              frame False {
              }
              frame True {
                # "nome do arquivo .cfg"
                # "seção no arquivo .cfg"
                # "open"
                n2761 = call-dynamic "Read Channel.vi"("error in (no error)"=w6115, "Acquisition in"=w6116) -> ("error out"=w6128:errorcluster, "Channel.lvclass"=w6129:refnum<class "Channel.lvclass">, "Acquisition out"=w6130:refnum<class "Acquisition.lvclass">)  [unwired: 7 in]
                n2762 = call-dynamic "Read Interface.vi"("error in (no error)"=w6128, "Channel in"=w6129) -> ("error out"=w6087:errorcluster, "Interface.lvclass"=w6088:refnum<class "Interface.lvclass">, "Channel out"=w6084:refnum<class "Channel.lvclass">)  [unwired: 7 in]
                n2763 = call-dynamic "Read restoreExpTime.vi"("error in (no error)"=w6087, "Interface in"=w6088) -> ("error out"=w6086:errorcluster, "restoreExpTime"=w6089:bool, "Interface out"=w6085:refnum<class "Interface.lvclass">)  [unwired: 7 in]
                n2764 = case shown="True" w6089 {
                  tunnel: w6085 -> [w6132 w6137]
                  tunnel: [w6132 w6140] -> w6093
                  tunnel: w6086 -> [w6131 w6136]
                  tunnel: [w6131 w6139] -> w6092
                  frame False {
                  }
                  frame True {
                    n2765 = call-dynamic "Write restoreExpTime.vi"("error in (no error)"=w6136, "restoreExpTime"=FALSE, "Interface in"=w6137) -> ("error out"=w6134:errorcluster, "Interface out"=w6135:refnum<class "Interface.lvclass">)  [unwired: 7 in]
                    n2766 = call-dynamic "Read prev ExpTime.vi"("error in (no error)"=w6134, "Interface in"=w6135) -> ("error out"=w6139:errorcluster, "prev ExpTime"=w6138:dbl, "Interface out"=w6140:refnum<class "Interface.lvclass">)  [unwired: 7 in]
                    n2767 = property on="Exptime ch4" class="DigNum (strict)"("Value"=w6138) -> ()  [unwired: 2 in, 2 out]
                  }
                }
                n2768 = call-dynamic "Read PREV_FT.vi"("error in (no error)"=w6092, "Interface in"=w6093) -> ("error out"=w6083:errorcluster, "PREV_FT"=w6094:bool, "Interface out"=w6081:refnum<class "Interface.lvclass">)  [unwired: 7 in]
                n2769 = call-dynamic "Read target cluster.vi"("error in (no error)"=w6083, "Channel in"=w6084) -> ("error out"=w6078:errorcluster, "target cluster"=w6082:T30, "Channel out"=w6080:refnum<class "Channel.lvclass">)  [unwired: 7 in]
                n2770 = Bundle By Name(cluster=w6082, "SHUTTER_MODE"=u8 1, "FRAME_TRANSFER"=w6094) -> (w6079:T30)
                n2771 = call-dynamic "Write target cluster.vi"("error in (no error)"=w6078, "target cluster"=w6079, "Channel in"=w6080) -> ("error out"=w6077:errorcluster, "Channel out"=w6076:refnum<class "Channel.lvclass">)  [unwired: 7 in]
                n2772 = Flatten To String(anything=w6079, error in (no error)=w6077) -> (data string=w6127:string, error out=w6126:errorcluster)  [unwired: 2 in, 1 out]
